vi "Delete Directory and SubDirectories.vi"(8 "error in (no error)":errorcluster caption="错误输入（无错误）", 10 "路径":path) -> (0 "error out":errorcluster caption="错误输出")   [LabVIEW 2012, in "Directory.lvclass"]
uses:
  Directory.lvclass
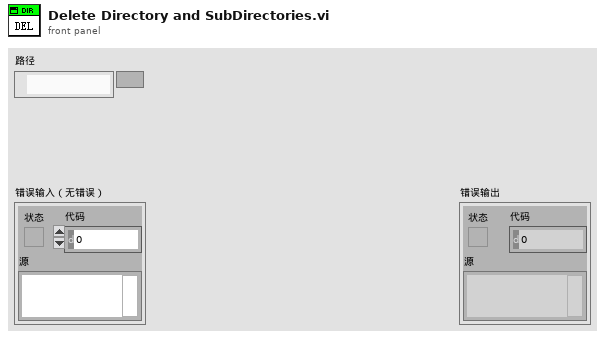
[diagram p1: front panel]
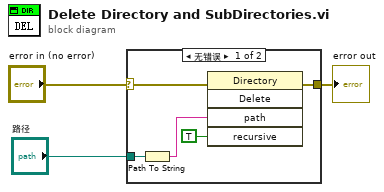
[diagram p0: block diagram]
diagram:
  n1 = case shown="无错误" "error in (no error)" {
    selector: "error in (no error)" -> [w8 w9]
    tunnel: [w7 w9] -> w2
    tunnel: "路径" -> [w6 _]
    frame No Error {
      n2 = Path To String(path=w6) -> (string=w5:string)
      n3 = invoke on="调用节点" class="Directory" method="Delete"(error in=w8, "path"=w5, "recursive"=TRUE) -> (error out=w7:errorcluster)  [unwired: 2 in, 4 out]
    }
    frame Error {
    }
  }
  "error out" <- w2
